vi "VII Pin Event Read Bytes.vi"(0 "DevType":i32, 1 "EventType":u16, 2 "SubAddr":u32, 3 "Len":u16, 5 "DevIndex":i32, 7 "I2CIndex":i32, 9 "EventPin":u16, 11 "error in (no error)":errorcluster, 12 "SlaveAddr":u16, 13 "pReadData":string, 14 "TimeOutMs":i32) -> (4 "pReadData out":string, 6 "function return":i32, 15 "error out":errorcluster)   [LabVIEW 2011, in "ControlI2C.lvlib"]
doc: "int __stdcall VII_PinEventReadBytes(int DevType,int DevIndex,int I2CIndex,unsigned short EventPin,unsigned short EventType,unsigned short SlaveAddr,unsigned int SubAddr,unsigned char* pReadData,unsigned short Len,int TimeOutMs);"
uses:
  ControlI2C.lvlib
  1234/Ginkgo_Driver.dll
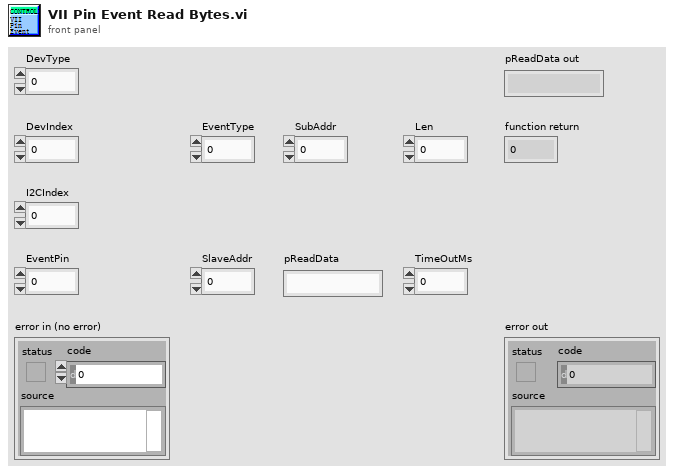
[diagram p1: front panel]
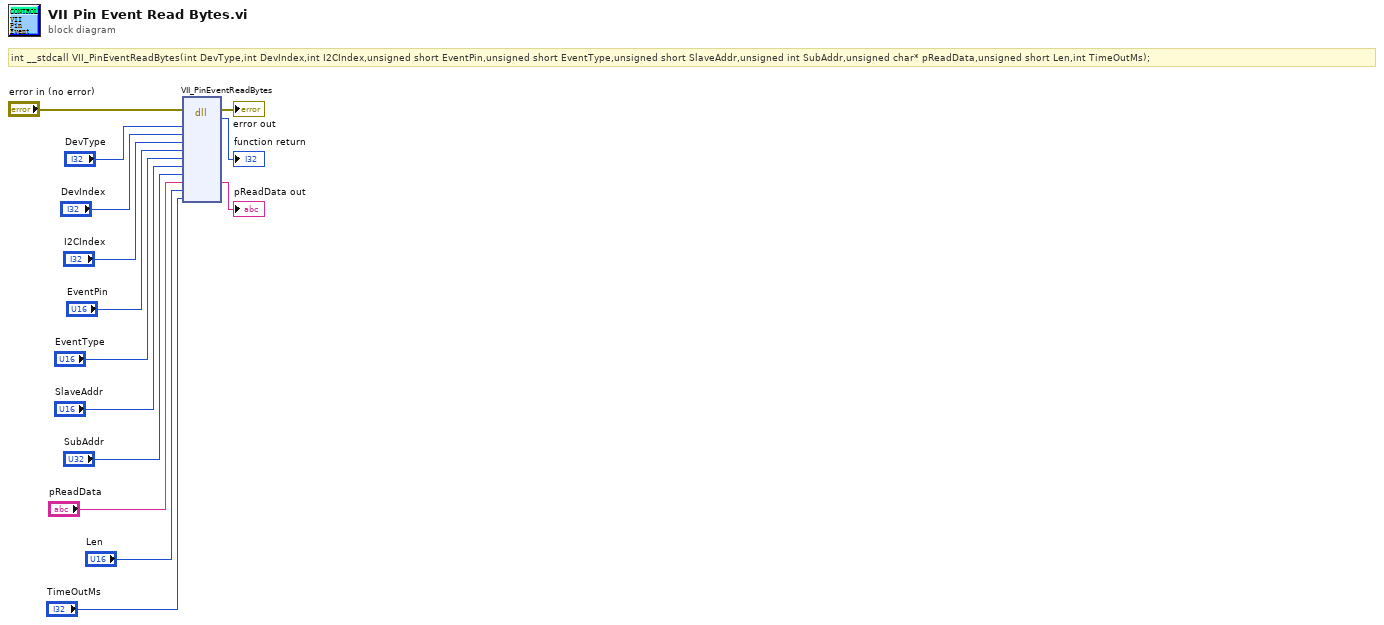
[diagram p0: block diagram]
diagram:
  # "int __stdcall VII_PinEventReadBytes(int DevType,int DevIndex,int I2CIndex,unsigned short EventPin,unsigned short EventType,unsigned short SlaveAddr,unsigned int SubAddr,unsigned char* pReadData,unsigned short Len,int TimeOutMs);"
  n1 = dll-call lib="E:/Project/vt_ginkgo/truck/Ginkgo Driver/vs2010/Ginkgo_USB-I2C&SPI&CAN_API_v2.0.3.3/lib/labview_32bit/1234/Ginkgo_Driver.*" fn="VII_PinEventReadBytes"(error in="error in (no error)", "DevType"="DevType", "DevIndex"="DevIndex", "I2CIndex"="I2CIndex", "EventPin"="EventPin", "EventType"="EventType", "SlaveAddr"="SlaveAddr", "SubAddr"="SubAddr", "pReadData"="pReadData", "Len"="Len", "TimeOutMs"="TimeOutMs") -> (error out=→"error out":errorcluster, →"function return":i32, "pReadData"=→"pReadData out":string)  [unwired: 11 in, 1 out]
